vi "staticcoord.vi"() -> ()   [LabVIEW 2012]
uses:
  <vilib>/vision/NI_Vision_Development_Module.lvlib
panel:
  out "String":string
  out "Image Out 2":T1(plugin-control)
  out "Image Out":T1(plugin-control)
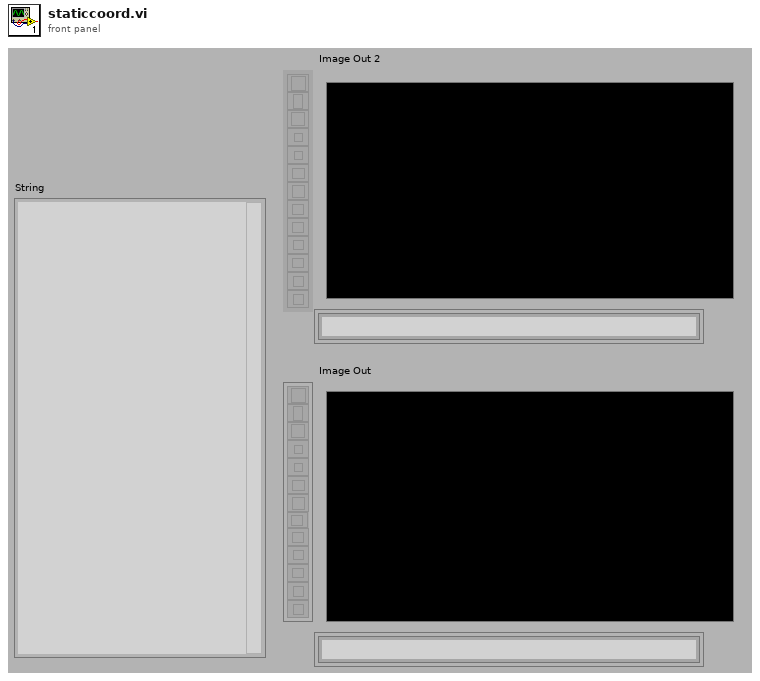
[diagram p1: front panel]
types:
  T1 = typedef "IMAQ Image.ctl" = refnum<image>
  T2 = cluster{"Object Center":cluster{"X":sgl, "Y":sgl}, "Bounding Box":cluster{"X Left":i32, "Y Top":i32, "X Right":i32, "Y Bottom":i32}, "Area":sgl, "Orientation":sgl, "Aspect Ratio":sgl, "Nb Holes":i32}[]
  T3 = cluster{"Object Center":cluster{"X":sgl, "Y":sgl}, "Bounding Box":cluster{"X Left":i32, "Y Top":i32, "X Right":i32, "Y Bottom":i32}, "Area":sgl, "Orientation":sgl, "Aspect Ratio":sgl, "Nb Holes":i32}
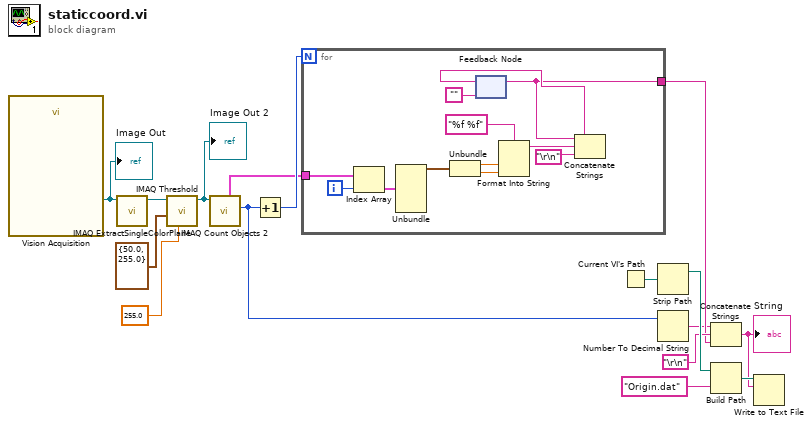
[diagram p0: block diagram]
diagram:
  n1 = call "Vision Acquisition"() -> ("Image Out"=w1:T1)  [unwired: 26 in, 1 out]
  "Image Out" <- w1
  n2 = call "IMAQ ExtractSingleColorPlane"("Image Src"=w1) -> ("Image Dst Out"=w14:T1)  [unwired: 9 in, 1 out]
  n3 = call "IMAQ Threshold"("Replace Value"=sgl 255.0 ("replace value"), "Range"=cluster{"lower value":sgl, "upper value":sgl} {"lower value"=50.0, "upper value"=255.0} ("threshold"), "Image Src"=w14) -> ("Image Dst Out"=w3:T1)  [unwired: 7 in, 1 out]
  "Image Out 2" <- w3
  n4 = call "IMAQ Count Objects 2"("Image"=w3) -> ("Number of Objects"=w2:i32, "Objects"=w4:T2)  [unwired: 6 in, 3 out]
  n5 = Increment(x=w2) -> (x+1=w8:i32)
  n6 = for {
    N: w8 -> [_]
    tunnel: w4 -> [w28]
    tunnel: [w20] -> w7
    i -> [w23]
    n7 = Index Array(array=w28, index=w23) -> (element=w27:T3)
    n8 = Unbundle(w27) -> ("Object Center"=w26:cluster{"X":sgl, "Y":sgl})  [unwired: 5 out]
    n9 = Unbundle(w26) -> ("X"=w17:sgl, "Y"=w18:sgl)
    n10 = feedback #1("") -> (w20:string)
    n11 = Format Into String(format string="%f %f", w17, w18) -> (resulting string=w22:string)  [unwired: 2 in, 1 out]
    n12 = Concatenate Strings(w20, w22, "\r\n") -> (w21:string)
    n13 = feedback-in #1(w21) -> ()
  }
  n14 = Current VI's Path() -> (path=w12:path)
  n15 = Strip Path(path=w12) -> (stripped path=w10:path)  [unwired: 1 out]
  n16 = Number To Decimal String(number=w2) -> (decimal integer string=w6:string)  [unwired: 1 in]
  n17 = Concatenate Strings(w6, "\r\n", w7) -> (w5:string)
  "String" <- w5
  n18 = Build Path(base path=w10, name or relative path="Origin.dat" ("standard input")) -> (appended path=w13:path)
  n19 = Write to Text File(file (use dialog)=w13, text=w5) -> ()  [unwired: 2 in, 3 out]
